vi "parse UHD XML.vi"() -> ()   [LabVIEW 2023]
uses:
  <vilib>/xml/Close Reference(Node).vi
  <vilib>/xml/NI_XML.lvlib
panel:
  out "size(s)":i32
  in  "base class":string
  out "error out":errorcluster
  out "Array":string[](array[string])
  in  "path to XML documents":path=path "C:/UHD/xml/classuhd_1_1rfnoc_1_1node__t.xml" caption="path to XML document"
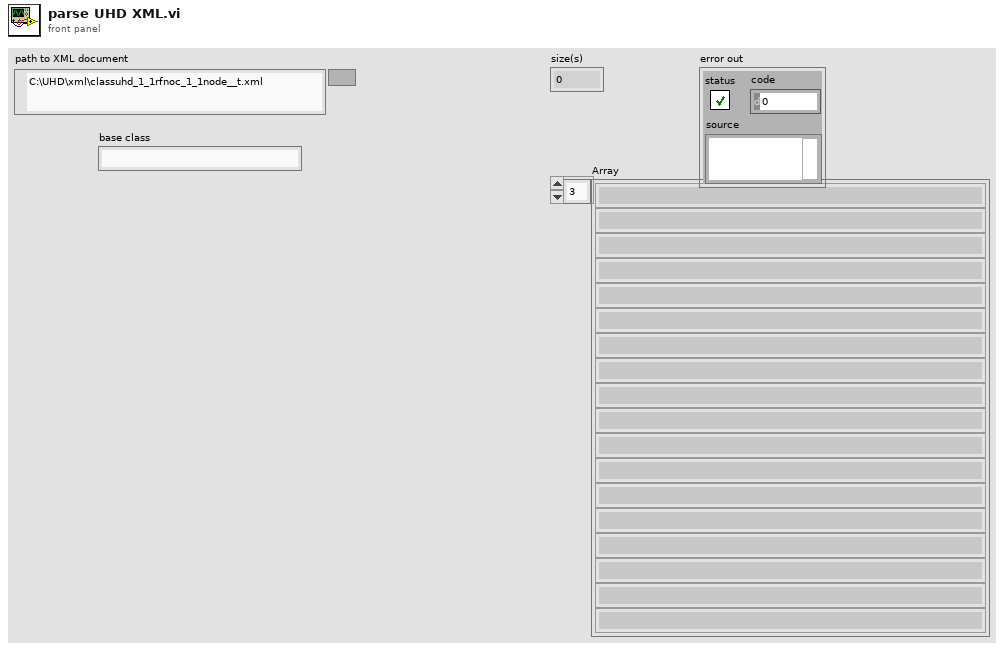
[diagram p1: front panel]
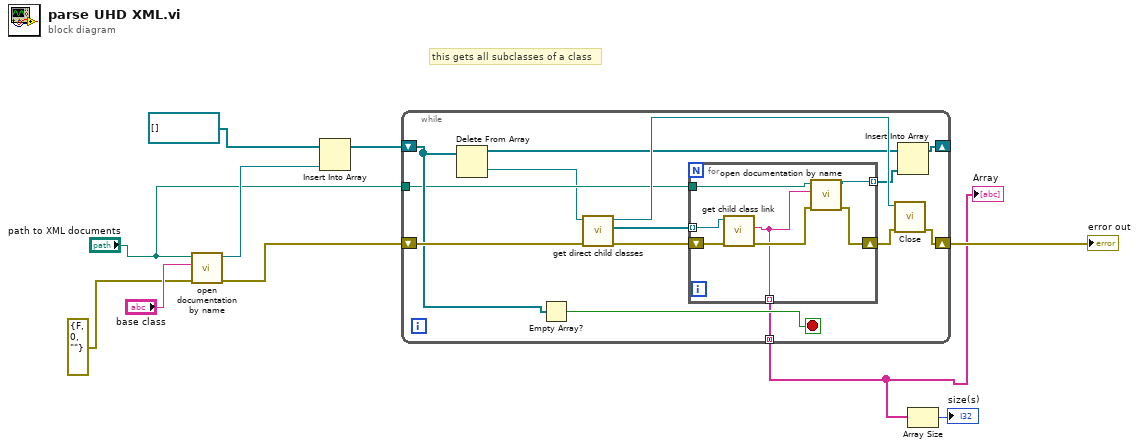
[diagram p0: block diagram]
diagram:
  # "this gets all subclasses of a class"
  n1 = call "open documentation by name.vi"("error in (no error)"=errorcluster {"status"=FALSE, "code"=0, "source"=""}, "base class"="base class", "path to XML documents"="path to XML documents") -> ("error out"=w10:errorcluster, "Refnum out"=w6:refnum<k20>)  [unwired: 7 in]
  n2 = Insert Into Array(array=refnum<k20>[] [] ("initialized array"), new element=w6) -> (w5:refnum<k20>[])  [unwired: 1 in]
  n3 = while {
    shift-right: [w18] -> w3
    shift-left: w10 -> [w24]
    shift-right: [w11] -> _
    shift-left: w5 -> [w20]
    tunnel: "path to XML documents" -> [w16]
    tunnel: [w14] -> w2 mode=concatenating
    stop <- w21 stop-if-true
    n4 = Delete From Array(array=w20) -> (deleted portion=w15:refnum<k20>, array with subset deleted=w13:refnum<k20>[])  [unwired: 2 in]
    n5 = Empty Array?(array=w20) -> (empty?=w21:bool)
    n6 = call "get direct child classes.vi"("error in (no error)"=w24, "node in"=w15) -> ("error out"=w23:errorcluster, "direct child classes"=w22:refnum<k20>[], "node out"=w17:refnum<k20>)  [unwired: 7 in]
    n7 = for {
      shift-right: [w27] -> w19
      shift-left: w23 -> [w31]
      tunnel: w22 -> [w30] mode=indexing
      tunnel: w16 -> [w29]
      tunnel: [w26] -> w12 mode=indexing
      tunnel: [w25] -> w14 mode=indexing
      n8 = call "get child class link.vi"("error in (no error)"=w31, "node in"=w30) -> ("error out"=w28:errorcluster, "link"=w25:string)  [unwired: 7 in, 1 out]
      n9 = call "open documentation by name.vi"("error in (no error)"=w28, "base class"=w25, "path to XML documents"=w29) -> ("error out"=w27:errorcluster, "Refnum out"=w26:refnum<k20>)  [unwired: 7 in]
    }
    n10 = call-poly <vilib>:"Close.vi"("error in (no error)"=w19, "node"=w17) -> ("error out"=w18:errorcluster)  [unwired: 7 in]
    n11 = Insert Into Array(array=w13, new element=w12) -> (w11:refnum<k20>[])  [unwired: 1 in]
  }
  "Array" <- w2
  "error out" <- w3
  n12 = Array Size(array=w2) -> (size(s)=→"size(s)":i32)
